vi "Calc_from-dT_dAng_to-dLaml.vi"() -> ()   [LabVIEW 2010]
uses:
  <vilib>/gmath/NI_Gmath.lvlib
panel:
  in  "Et T(K) 2":dbl=56.5
  in  "Angle (deg) 2":dbl=5.0 format="%.3f"
  out "dV to angle to":dbl=-2.1315141762734413e-07 format="%.1f"
  out "dV to 0 deg":dbl=-2.1315141762734413e-07 format="%.1f"
  out "d l @ angle to":dbl format="%_6g"
  in  "Angle to (deg)":dbl=5.0 format="%.3f"
  out "d l  @ max angle":dbl=-2.1315141762734413e-07 format="%_6g"
  out "d l  @ 0 deg":dbl=1.1354370466065689e-07 format="%_6g"
  in  "Et thickness":dbl=210.0 format="%.1f"
  in  "Wavelength":dbl=1.21 format="%_6g"
  out "Temperature vs refractive index":cluster{"Refr index raw":dbl[], "yi":dbl[]}[](graph)=[{"Refr index raw"=[3.51113, 3.51123, 3.51146, 3.51181, 3.51229, 3.51288, 3.51358, 3.51439, 3.51979, 3.52703, 3.53555, 3.54394], "yi"=[30.0, 40.0, 50.0, 60.0, 70.0, 80.0, 90.0, 100.0, 150.0, 200.0, 250.0, 295.0]}, {"Refr index raw"=[3.511673627651122], "yi"=[56.528812518598016]}]
  out "refr inx master from":dbl=3.511673627651122
  in  "Et T(K) 1":dbl=56.5
  out "dV to max angle":dbl=-2.1315141762734413e-07 format="%.1f"
  in  "Angle (deg) 1":dbl=5.0 format="%.3f"
  out "Out of  Range":bool
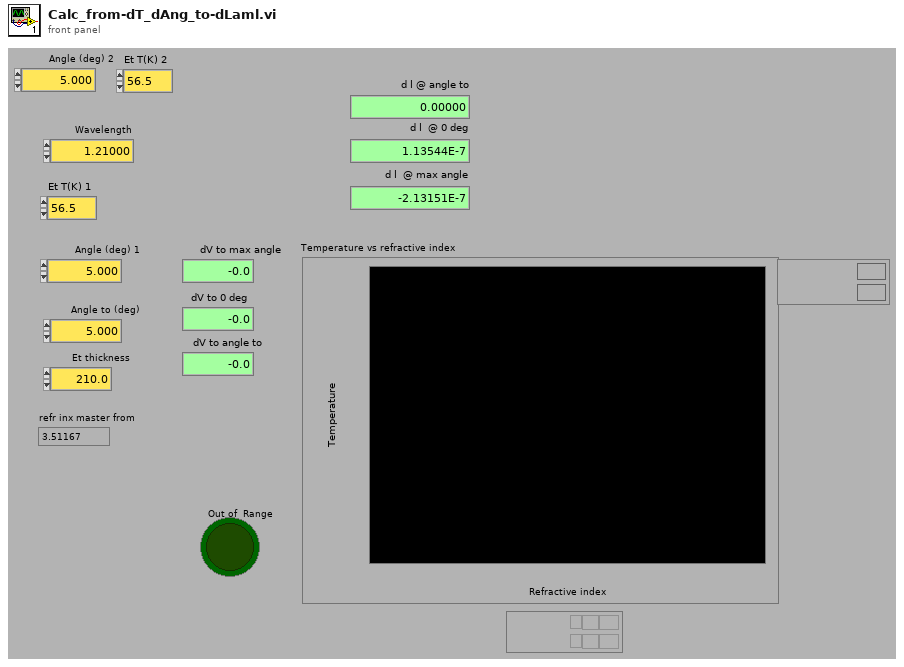
[diagram p1: front panel]
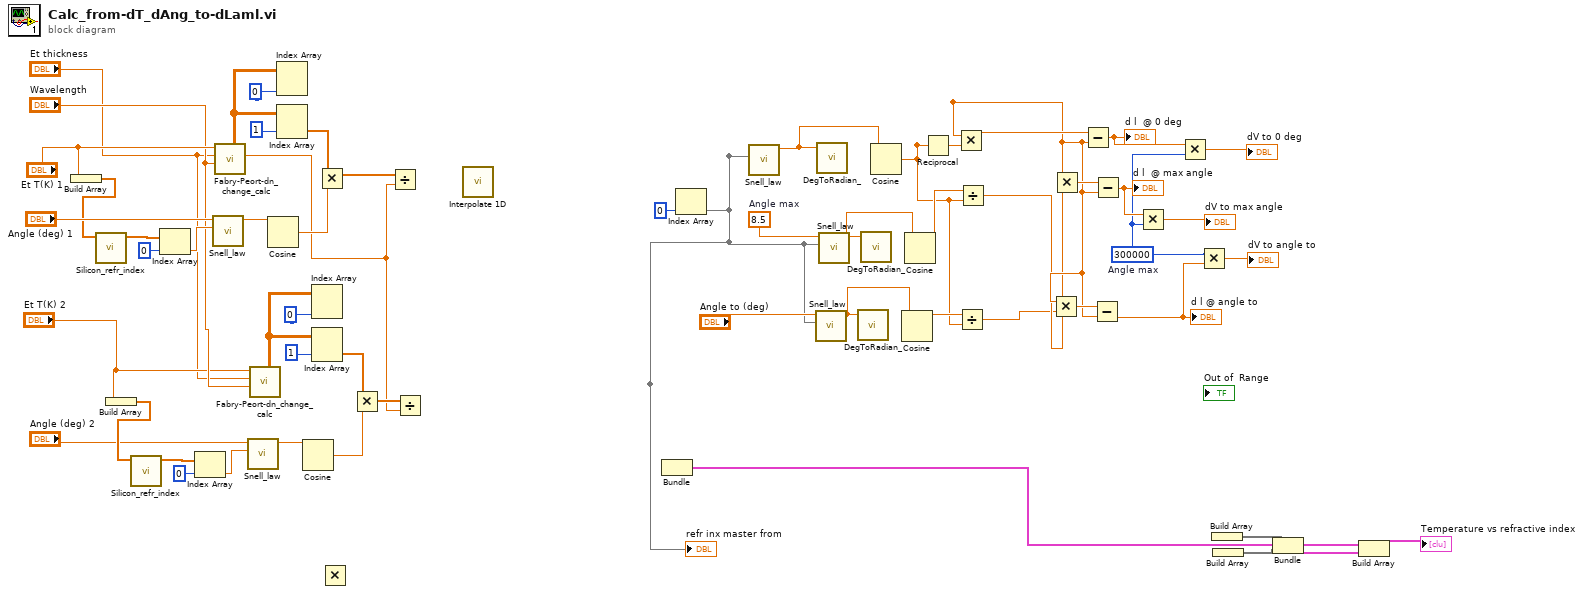
[diagram p0: block diagram]
diagram:
  w34 = 300000  # Angle max
  w55 = 8.5  # Angle max
  n1 = Build Array("Et T(K) 1") -> (w27:dbl[])
  n2 = call "Silicon_refr_index.vi"("Temperature"=w27) -> ("Silicon refr index at T"=w25:dbl[])  [unwired: 8 in, 2 out]
  n3 = Build Array("Et T(K) 2") -> (w8:dbl[])
  n4 = call "Silicon_refr_index.vi"("Temperature"=w8) -> ("Silicon refr index at T"=w10:dbl[])  [unwired: 8 in, 2 out]
  n5 = Index Array(array=w25, index=0) -> (element=w24:dbl)
  n6 = Index Array(array=w10, index=0) -> (element=w11:dbl)
  n7 = call "Snell_law.vi"("Refr index"=w24, "Angle in ext (deg)"="Angle (deg) 1") -> ("Angle out int (rad)"=w23:dbl)  [unwired: 8 in, 1 out]
  n8 = call "Fabry-Peort-dn_change_calc.vi"("Wavelength"="Wavelength", "Et thickness at 300K"="Et thickness", "Et T(K)  initial"="Et T(K) 1") -> ("Order"=w1:dbl, "T and dn arr"=w20:dbl[][])  [unwired: 4 in, 3 out]
  n9 = call "Snell_law.vi"("Refr index"=w11, "Angle in ext (deg)"="Angle (deg) 2") -> ("Angle out int (rad)"=w12:dbl)  [unwired: 8 in, 1 out]
  n10 = call "Fabry-Peort-dn_change_calc.vi"("Wavelength"="Wavelength", "Et thickness at 300K"="Et thickness", "Et T(K)  initial"="Et T(K) 2") -> ("T and dn arr"=w15:dbl[][])  [unwired: 4 in, 4 out]
  n11 = Cosine(x=w23) -> (cos(x)=w18:dbl)
  n12 = Index Array(array=w20, index (col)=0 ("index")) -> ()  [unwired: 1 in, 1 out]
  n13 = Index Array(array=w20, index (col)=1 ("index")) -> (element=w19:dbl[])  [unwired: 1 in]
  n14 = Cosine(x=w12) -> (cos(x)=w17:dbl)
  n15 = Index Array(array=w15, index (col)=0 ("index")) -> ()  [unwired: 1 in, 1 out]
  n16 = Index Array(array=w15, index (col)=1 ("index")) -> (element=w16:dbl[])  [unwired: 1 in]
  n17 = Multiply(x=w19, y=w18) -> (x*y=w3:dbl[])
  n18 = Multiply() -> ()  [unwired: 2 in, 1 out]
  n19 = Multiply(x=w16, y=w17) -> (x*y=w2:dbl[])
  n20 = Divide(x=w3, y=w1) -> ()  [unwired: 1 out]
  n21 = Divide(x=w2, y=w1) -> ()  [unwired: 1 out]
  n22 = call <vilib>:"Interpolate 1D.vi"() -> ()  [unwired: 9 in, 3 out]
  n23 = Bundle() -> (w43:cluster{void, void}, w62, w61)  [unwired: 1 in]
  n24 = Index Array(index=0) -> (array=w58:dbl[], element=w30)
  "refr inx master from" <- w30
  n25 = call "Snell_law.vi"("Refr index"=w30) -> ("Angle out int (rad)"=w42:dbl)  [unwired: 9 in, 1 out]
  n26 = call "Snell_law.vi"("Refr index"=w30, "Angle in ext (deg)"="Angle to (deg)") -> ("Angle out int (rad)"=w41:dbl)  [unwired: 8 in, 1 out]
  n27 = call "DegToRadian_.vi"("Angle deg"=w42) -> ()  [unwired: 4 in, 1 out]
  n28 = call "Snell_law.vi"("Refr index"=w30, "Angle in ext (deg)"=w55) -> ("Angle out int (rad)"=w40:dbl)  [unwired: 8 in, 1 out]
  n29 = call "DegToRadian_.vi"("Angle deg"=w41) -> ()  [unwired: 4 in, 1 out]
  n30 = call "DegToRadian_.vi"("Angle deg"=w40) -> ()  [unwired: 4 in, 1 out]
  n31 = Cosine(x=w42) -> (cos(x)=w32:dbl)
  n32 = Cosine(x=w41) -> (cos(x)=w48:dbl)
  n33 = Cosine(x=w40) -> (cos(x)=w54:dbl)
  n34 = Reciprocal(x=w32) -> (1/x=w46:dbl)
  n35 = Divide(x=w48, y=w32) -> (x/y=w31:dbl)
  n36 = Divide(x=w54, y=w32) -> (x/y=w47:dbl)
  n37 = Multiply(y=w47) -> (x=w49:dbl, x*y=w52:dbl)
  n38 = Multiply(x=w49, y=w46) -> (x*y=w53:dbl)
  n39 = Multiply(x=w49, y=w31) -> (x*y=w50:dbl)
  n40 = Subtract(x=w53, y=w49) -> (x-y=w37:dbl)
  "d l  @ 0 deg" <- w37
  n41 = Subtract(x=w50, y=w49) -> (x-y=w35:dbl)
  "d l @ angle to" <- w35
  n42 = Subtract(x=w52, y=w49) -> (x-y=w39:dbl)
  "d l  @ max angle" <- w39
  n43 = Multiply(x=w39, y=w34) -> (x*y=→"dV to max angle":dbl)
  n44 = Multiply(x=w37, y=w34) -> (x*y=→"dV to 0 deg":dbl)
  n45 = Multiply(x=w34, y=w35) -> (x*y=→"dV to angle to":dbl)
  n46 = Build Array() -> (w59:void[], w44:dbl)
  n47 = Build Array() -> (w60:void[], w45:dbl)
  n48 = Bundle(w59, w60) -> (w63:cluster{void[], void[]})  [unwired: 1 in]
  n49 = Build Array(w43, w63) -> (→"Temperature vs refractive index":cluster{void[], void[]}[])
